vi "Create_Object.vi"(8 "error in (no error)":errorcluster, 9 "Block Diagram in":T1, 10 "owner refnum":variant, 11 "String Constant in":refnum<class "String Constant.lvclass">) -> (0 "error out":errorcluster, 1 "Block Diagram Out":T1, 3 "String Constant out":refnum<class "String Constant.lvclass">)   [LabVIEW 2025, in "String Constant.lvclass"]
uses:
  String Constant.lvclass
  C:/Users/mrjak/Documents/GitHub/LVGPT/LabVIEW/VIs/Classes/Node/Node.lvclass
  Controls/bd.ctl
  Node.lvclass
  Controls/wire.ctl
  Controls/Terminal.ctl
  Node.lvclass/Node.ctl
  Constant.lvclass
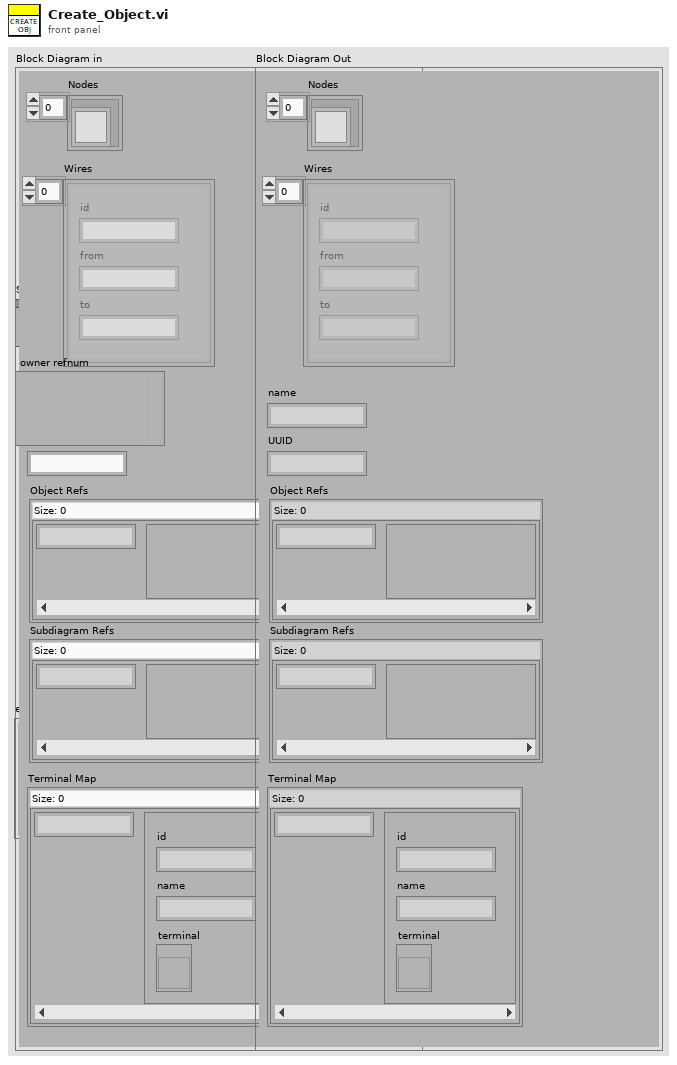
[diagram p1: front panel]
types:
  T1 = typedef "bd.ctl" = cluster{"Nodes":refnum<class "Node.lvclass">[], "Wires":T2[], "name":string, "UUID":string, "Object Refs":map{string, variant}, "Subdiagram Refs":map{string, variant}, "Terminal Map":map{string, T3}}
  T2 = typedef "wire.ctl" = cluster{"id":string, "from":string, "to":string}
  T3 = typedef "Terminal.ctl" = cluster{"id":string, "name":string, "terminal":refnum<vi>}
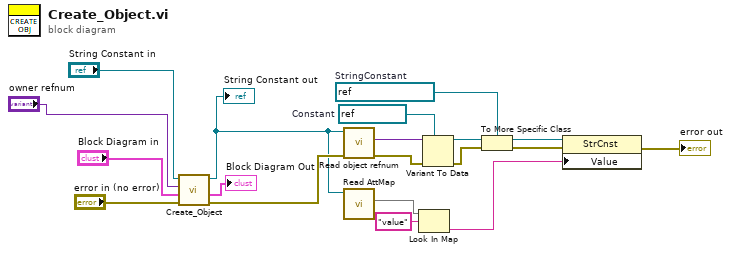
[diagram p0: block diagram]
diagram:
  w11 = refnum<vi> refnum  # StringConstant
  w13 = refnum<vi> refnum  # Constant
  n1 = call-parent "Create_Object.vi"("error in (no error)"="error in (no error)", "Block Diagram in"="Block Diagram in", "owner refnum"="owner refnum", "Constant in"="String Constant in") -> ("error out"=w16:errorcluster, "Block Diagram Out"=→"Block Diagram Out":T1, "Constant out"=w3:refnum<class "String Constant.lvclass">)  [unwired: 5 in]
  "String Constant out" <- w3
  n2 = call-dynamic "Read object refnum.vi"("error in (no error)"=w16, "Node in"=w3) -> ("error out"=w10:errorcluster, "object refnum"=w14:variant)  [unwired: 7 in, 1 out]
  n3 = call "Read AttMap.vi"("Node in"=w3) -> ("AttMap"=w6:map{string, string})  [unwired: 8 in, 2 out]
  n4 = Look In Map(map=w6, key="value") -> (value=w4:string)  [unwired: 1 in, 1 out]
  n5 = Variant To Data(error in=w10, type=w13, Variant=w14) -> (data=w12:refnum<vi>, error out=w9:errorcluster)
  n6 = To More Specific Class(target class=w11, reference=w12, error in=w9) -> (specific class reference=w8:refnum<vi>, error out=w7:errorcluster)
  n7 = property class="StrCnst"(reference=w8, error in=w7, "Value"=w4) -> (error out=→"error out":errorcluster)  [unwired: 1 out]
